vi "getControlData.vi"(11 "system matricec path":path=path "C:/Users/arnold/Documents/MATLAB/AFM_statespace/data/exp01Controls.csv") -> (2 "AllMatrix":dbl[](array[numeric]), 3 "controlParams":T1={"NS"=7, "ND"=10, "Nbar"=1.253469179440319, "Ki"=0.125346917944, "ref"=0.125346917944} {"ref" format="%#_13g"; "Ki" format="%#_13g"; "Nbar" format="%#_13g"})   [LabVIEW 2017]
uses:
  controls/ControlParams.ctl
  <vilib>/Utility/file.llb/Read From Spreadsheet File (DBL).vi
panel:
  in  "Cluster":T1={"NS"=7, "ND"=10, "Nbar"=1.253469179440319, "Ki"=0.125346917944, "ref"=0.125346917944} {"ref" format="%#_13g"; "Ki" format="%#_13g"; "Nbar" format="%#_13g"}
  # "This vi gets control data from a .csv file. It expects the data in\nthe following format:\n| B,   Ki       |\n| L,    Nbar |\n|K',   Ns      |\n|C',   Nd     |\n|Arn,  ref    |\n|.         0      |\n|.         0      |"
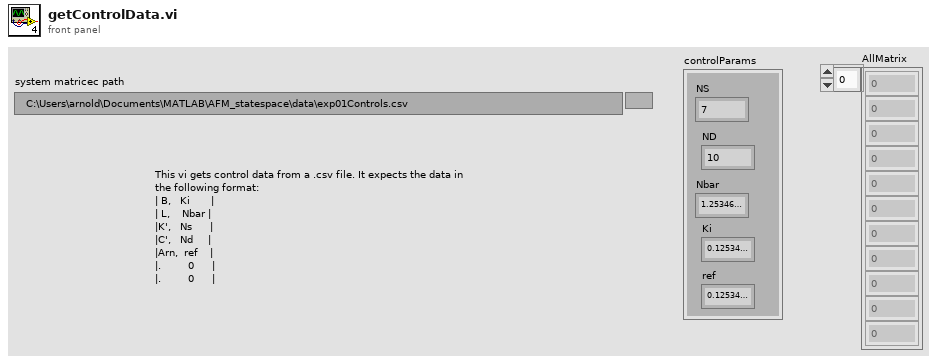
[diagram p1: front panel]
types:
  T1 = typedef "ControlParams.ctl" = cluster{"NS":i32, "ND":i32, "Nbar":dbl, "Ki":dbl, "ref":dbl}
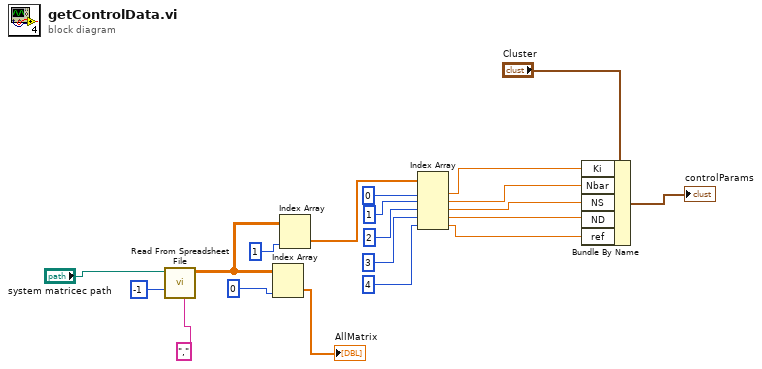
[diagram p0: block diagram]
diagram:
  n1 = call-poly <vilib>:"Read From Spreadsheet File.vi"("delimiter (\\t)"=",", "number of rows (all:-1)"=-1, "file path (dialog if empty)"="system matricec path") -> ("all rows"=w6:dbl[][])  [unwired: 4 in, 4 out]
  n2 = Index Array(array=w6, index (col)=0 ("dimension size")) -> (element=→"AllMatrix":dbl[])  [unwired: 1 in]
  n3 = Index Array(array=w6, index (col)=1 ("dimension size")) -> (element=w10:dbl[])  [unwired: 1 in]
  n4 = Index Array(array=w10, index #1=0, index #2=1, index #3=2, index #4=3, index #5=4) -> (element #1=w12:dbl, element #2=w13:dbl, element #3=w14:dbl, element #4=w15:dbl, element #5=w1:dbl)
  n5 = Bundle By Name(cluster="Cluster", "Ki"=w12, "Nbar"=w13, "NS"=w14, "ND"=w15, "ref"=w1) -> (→"controlParams":T1)
